vi "Wait on Server Loop.vi"(8 "error in (no error)":errorcluster, 10 "Value":bool, 11 "TCP Server in":refnum<class "TCP Server.lvclass">) -> (0 "error out":errorcluster, 3 "TCP Server out":refnum<class "TCP Server.lvclass">)   [LabVIEW 2020, in "Stream-TCP.lvlib" / "TCP Server.lvclass"]
uses:
  TCP Server.lvclass
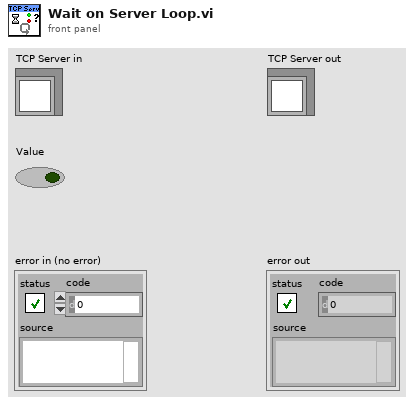
[diagram p1: front panel]
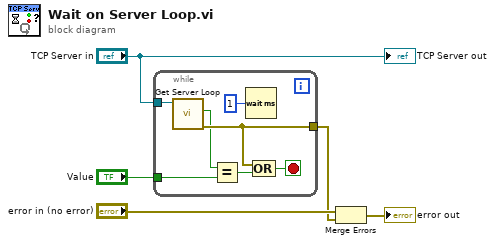
[diagram p0: block diagram]
diagram:
  n1 = while {
    tunnel: "Value" -> [w12]
    tunnel: [w7] -> w3
    tunnel: "TCP Server in" -> [w8]
    stop <- w10 stop-if-true
    n2 = call "Get Server Loop.vi"("TCP Server in"=w8) -> ("error out"=w7:errorcluster, "Server Loop"=w6:bool)  [unwired: 8 in, 1 out]
    n3 = Equal?(x=w6, y=w12) -> (x = y?=w11:bool)
    n4 = Wait (ms)(milliseconds to wait=u32 1) -> ()  [unwired: 1 out]
    n5 = Compound Arithmetic op=OR(w7, w11) -> (w10:bool)
  }
  n6 = Merge Errors("error in (no error)", w3) -> (→"error out":errorcluster)
  "TCP Server out" <- "TCP Server in"
